vi "Model Selection.vi"() -> ()   [LabVIEW 2018]
panel:
  in  "MODEL IN":enum16{"E183362", "E180639", "E415025"}(ring)
  in  "MODEL":enum16{"E183362", "E180639", "E415025"}(ring)
  in  "ME79MODEL":bool
  in  "Model":bool
  in  "CANCEL":bool
  in  "OK":bool
  in  "ME79Model":bool
  in  "Model":bool
  # "PLEASE SELECT MODEL"
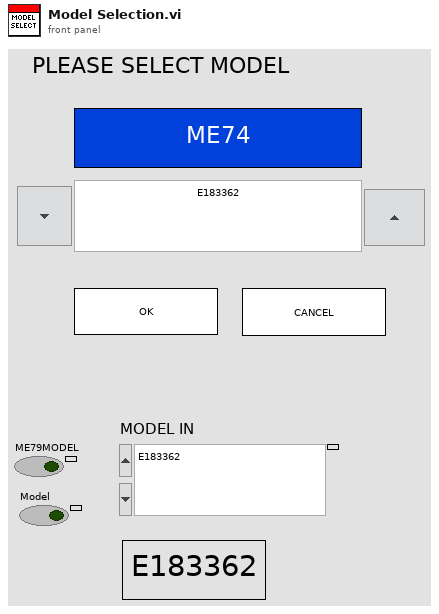
[diagram p1: front panel]
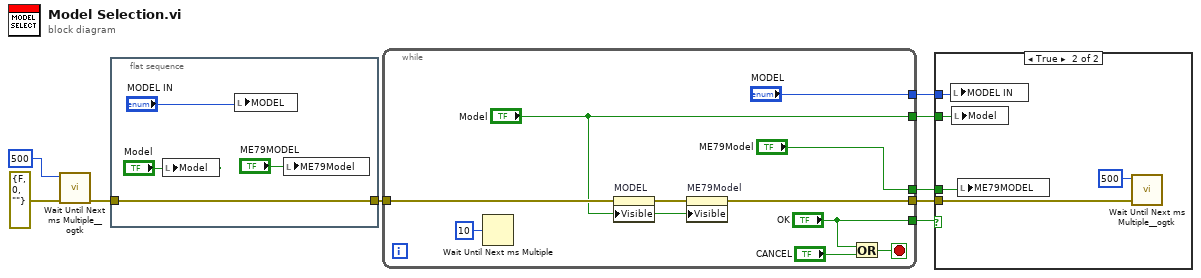
[diagram p0: block diagram]
diagram:
  n1 = call <userlib>:"Wait Until Next ms Multiple__ogtk.vi"("error in (no error)"=errorcluster {"status"=FALSE, "code"=0, "source"=""}, "milliseconds to wait"=u32 500) -> ("error out"=w4:errorcluster)  [unwired: 8 in, 1 out]
  n2 = flat-sequence {
    tunnel: [w13] -> w5
    tunnel: w4 -> [w13]
    frame #0 {
      n3 = local write "Model"("Model") -> ()
      n4 = local write "MODEL"("MODEL IN") -> ()
      n5 = local write "ME79Model"("ME79MODEL") -> ()
    }
  }
  n6 = while {
    tunnel: w5 -> [w17]
    tunnel: ["ME79Model"] -> w8
    tunnel: ["Model"] -> w7
    tunnel: ["OK"] -> w9
    tunnel: [w19] -> w6
    tunnel: ["MODEL"] -> w1
    stop <- w21 stop-if-true
    n7 = Wait Until Next ms Multiple(millisecond multiple=u32 10) -> ()  [unwired: 1 out]
    n8 = property on="MODEL" class="Enum (strict)"(error in=w17, "Visible"="Model") -> (error out=w16:errorcluster)  [unwired: 1 in, 1 out]
    n9 = property on="ME79Model" class="Bool (strict)"(error in=w16, "Visible"="Model") -> (error out=w19:errorcluster)  [unwired: 1 in, 1 out]
    n10 = Or(x="OK", y="CANCEL") -> (x .or. y?=w21:bool)
  }
  n11 = case shown="True" w9 {
    tunnel: w8 -> [_ w27]
    tunnel: w7 -> [_ w26]
    tunnel: w6 -> [_ w28]
    tunnel: w1 -> [_ w24]
    frame False {
    }
    frame True {
      n12 = local write "MODEL IN"(w24) -> ()
      n13 = local write "Model"(w26) -> ()
      n14 = local write "ME79MODEL"(w27) -> ()
      n15 = call <userlib>:"Wait Until Next ms Multiple__ogtk.vi"("error in (no error)"=w28, "milliseconds to wait"=u32 500) -> ()  [unwired: 8 in, 2 out]
    }
  }
